vi "ParameterOptimizationCalibration.vi"() -> ()   [LabVIEW 2020]
uses:
  <vilib>/silver_ctls/ArrayMatrixCluster/Real Matrix NI_Silver.ctl
  <vilib>/gmath/GlobalOptimization.llb/DE_Settings.ctl
  <vilib>/gmath/GlobalOptimization.llb/DE_Bound Mapping Method.ctl
  <vilib>/gmath/GlobalOptimization.llb/DE_Mutation Method.ctl
  <vilib>/gmath/GlobalOptimization.llb/DE_Crossover Method.ctl
  <vilib>/gmath/GlobalOptimization.llb/DE_Stopping Criteria.ctl
  <vilib>/gmath/GlobalOptimization.llb/DE_State.ctl
  <vilib>/gmath/GlobalOptimization.llb/DE_Population.ctl
  <vilib>/gmath/NI_AAL_GlobalOptimization.lvlib
panel:
  out "number of function calls":i32
  out "Minimum":dbl[](array[numeric])
  out "F(Minimum)":dbl[](array[numeric])
  in  "Beginning State":T1
  in  "stopping criteria":T3={"max iterations"=50, "max function calls"=-1, "max time (sec)"=-1.0}
  in  "DE settings":T4={"population size"=10, "scale factor"=0.9, "crossover probability"=0.95, "bound mapping method"=1, "mutation method"=0, "crossover method"=0} {"crossover method" items=["Uniform", "Exponential"]; "mutation method" items=["Random", "Either Or", "Best", "Target to Best"]; "bound mapping method" items=["None", "Random between Bounds and Values", "Re-Initialize"]}
  out "min index(es)":i32[](array[numeric])
  out "min value":dbl
  out "Intensity Graph":dbl[][](graph)
  in  "P(x)":dbl[](array[numeric])=[-0.407, 0.781, 0.000845, -0.0056] step=1e-10 format="%#.8f"
  out "Real Matrix":T8
  in  "Offset (D)":dbl[](array[numeric])=[-0.4, -0.5, 2.0, 3.0, 4.0]
  in  "C parameter":dbl[](array[numeric])=[0.0, 1.0, 2.0, 3.0, 4.0]
  out "Measured":waveform(dbl)(graph)={"t0"=timestamp(0 s since 1904-01-01), "dt"=1.0, "Y"=array[3075 elements]}
  out "error":waveform(dbl)(graph)={"t0"=timestamp(0 s since 1904-01-01), "dt"=1.0, "Y"=array[3075 elements]}
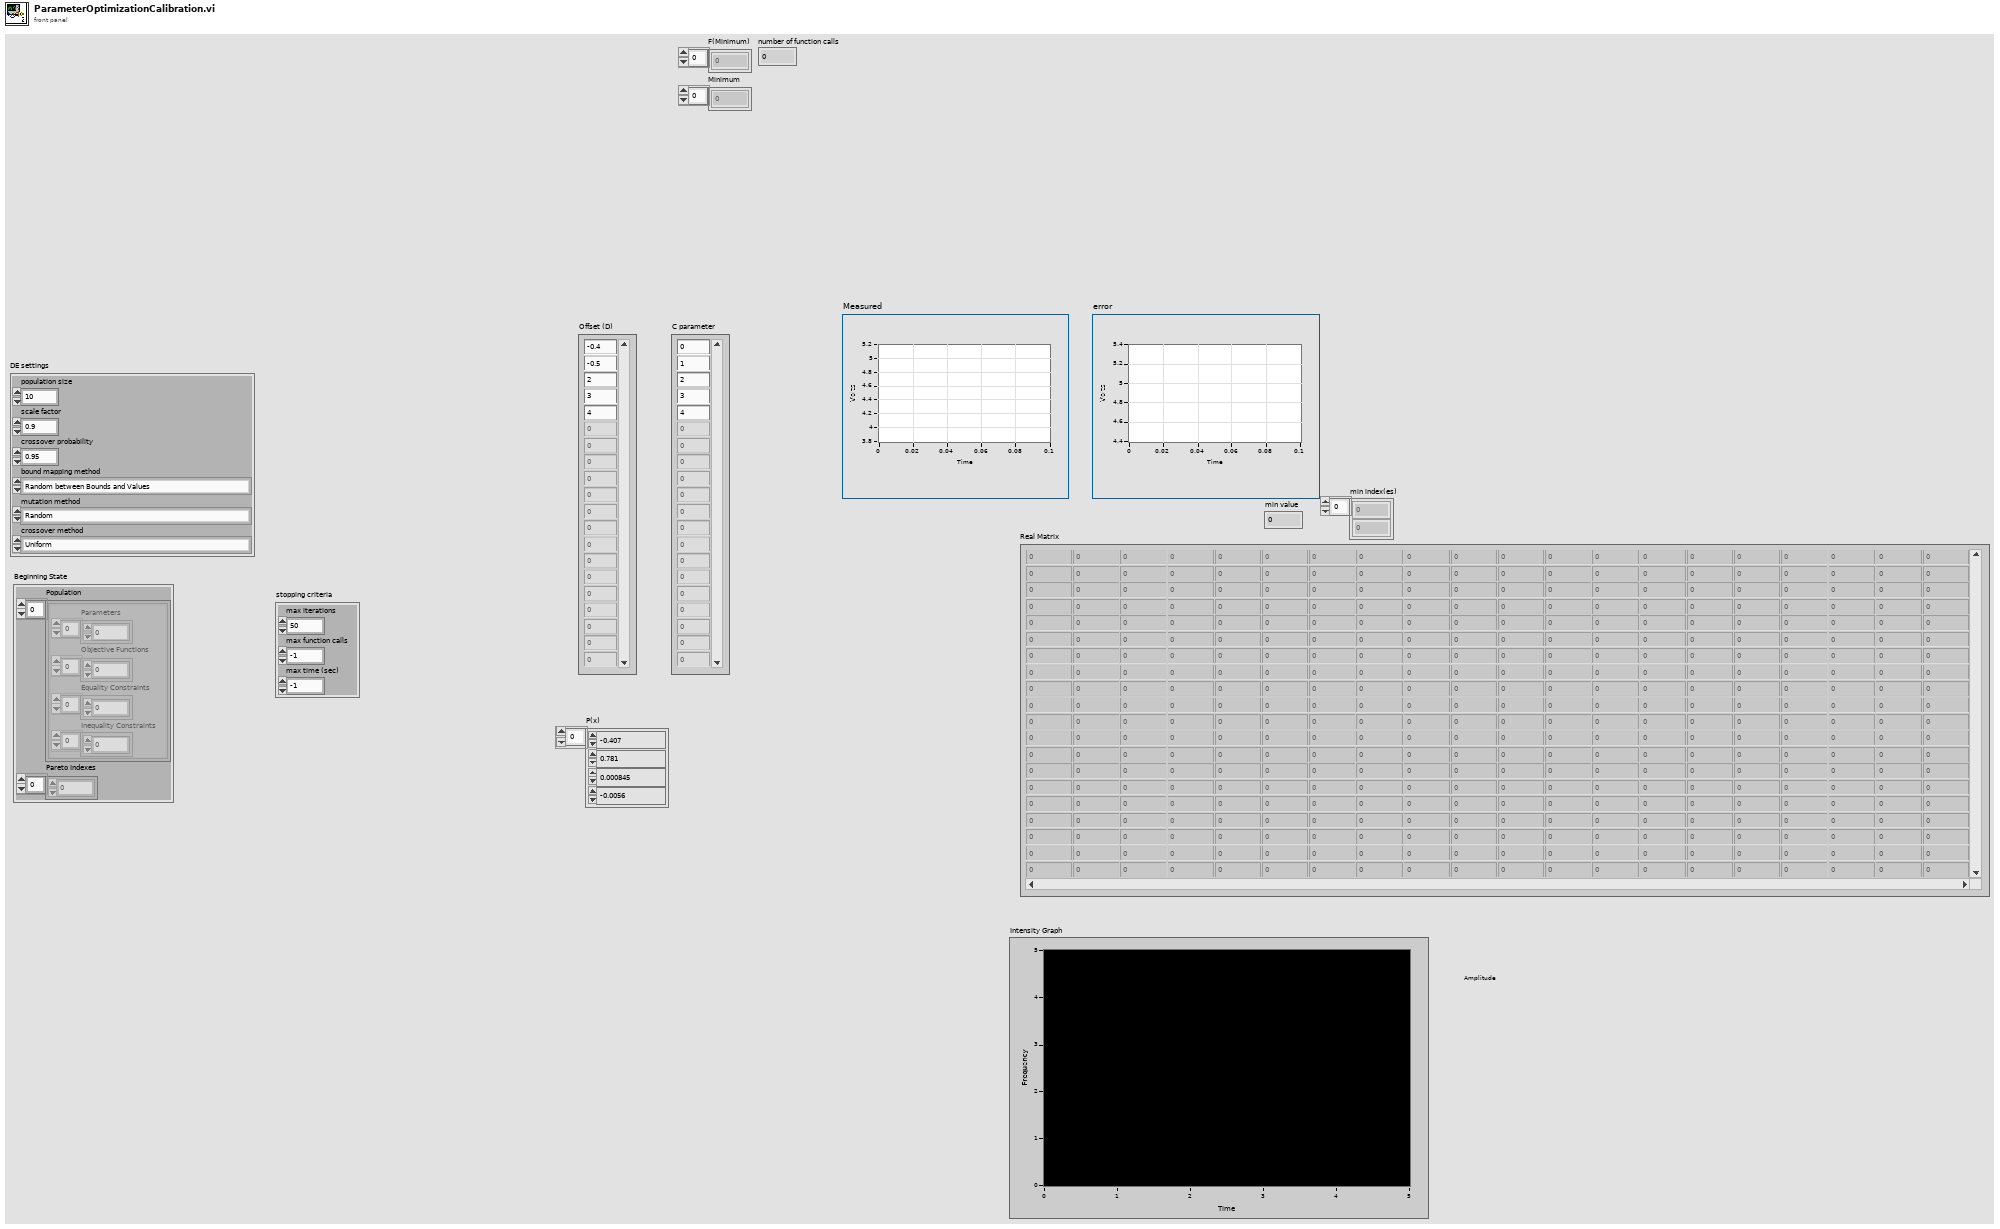
[diagram p1: front panel]
types:
  T1 = typedef "NI_AAL_GlobalOptimization.lvlib/DE_State.ctl" = cluster{"Population":T2[], "Pareto Indexes":i32[]}
  T2 = typedef "NI_AAL_GlobalOptimization.lvlib/DE_Population.ctl" = cluster{"Parameters":dbl[], "Objective Functions":dbl[], "Equality Constraints":dbl[], "Inequality Constraints":dbl[]}
  T3 = typedef "NI_AAL_GlobalOptimization.lvlib/DE_Stopping Criteria.ctl" = cluster{"max iterations":i32, "max function calls":i32, "max time (sec)":dbl}
  T4 = typedef "NI_AAL_GlobalOptimization.lvlib/DE_Settings.ctl" = cluster{"population size":i32, "scale factor":dbl, "crossover probability":dbl, "bound mapping method":T5, "mutation method":T6, "crossover method":T7}
  T5 = typedef "NI_AAL_GlobalOptimization.lvlib/DE_Bound Mapping Method.ctl" = u16
  T6 = typedef "NI_AAL_GlobalOptimization.lvlib/DE_Mutation Method.ctl" = u16
  T7 = typedef "NI_AAL_GlobalOptimization.lvlib/DE_Crossover Method.ctl" = u16
  T8 = typedef "Real Matrix NI_Silver.ctl" = dbl[][]
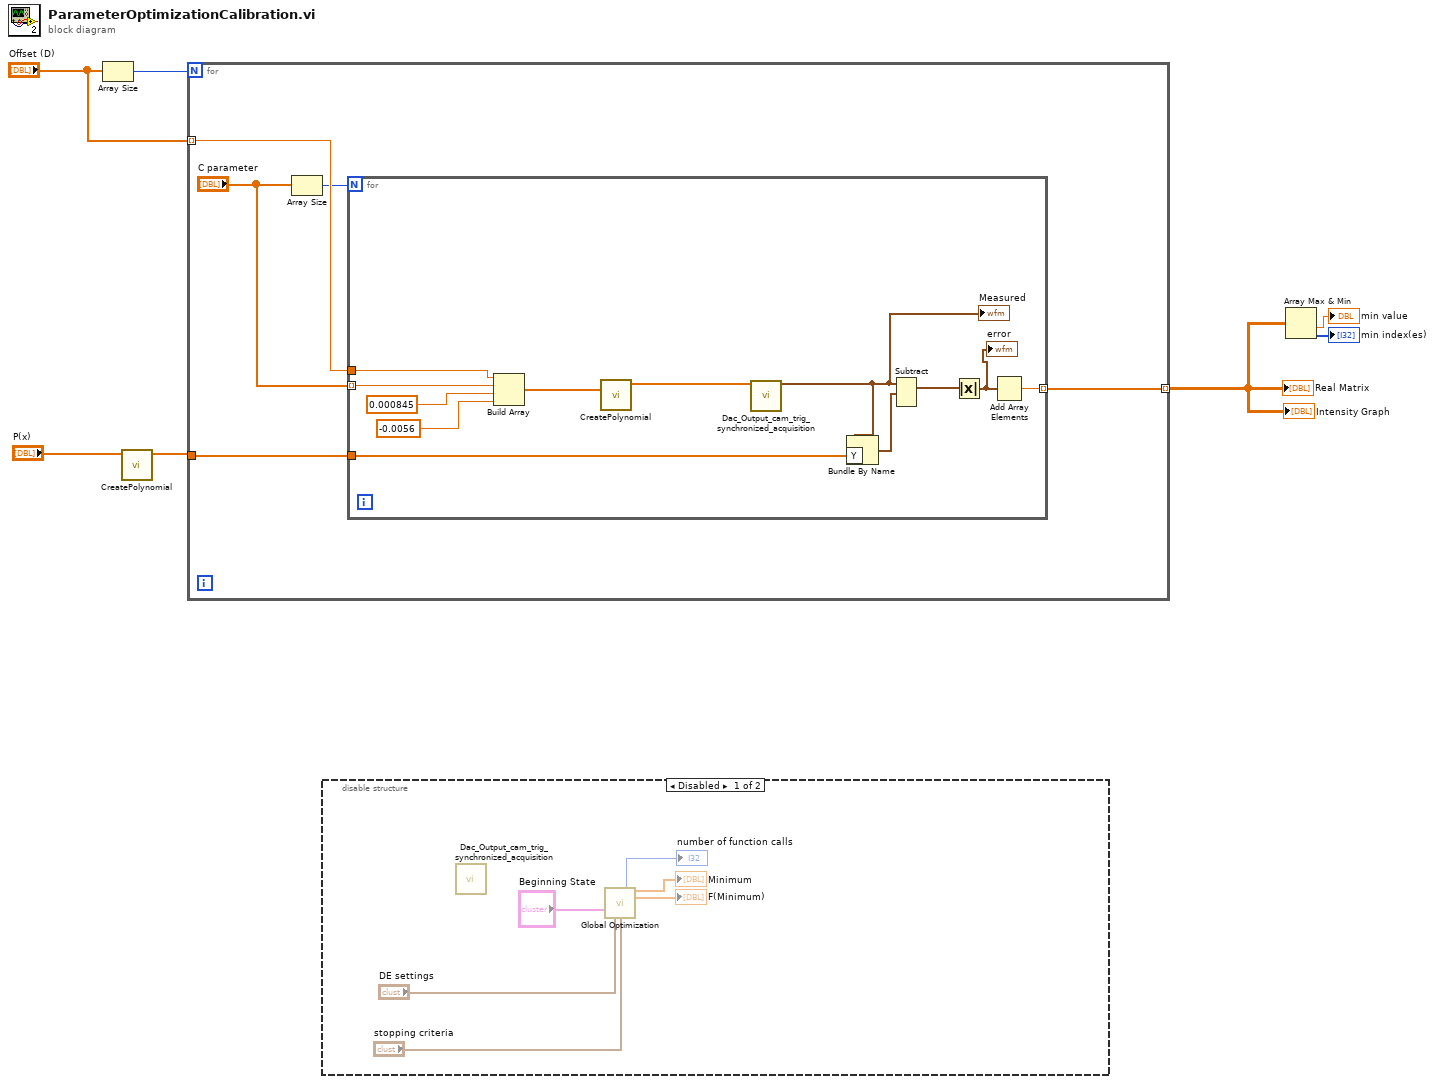
[diagram p0: block diagram]
diagram:
  n1 = Array Size(array="Offset (D)") -> (size(s)=w7:i32)
  n2 = call "CreatePolynomial.vi"("P(x)"="P(x)") -> ("Waveform Graph"=w4:dbl[])  [unwired: 9 in]
  n3 = for {
    N: w7 -> [_]
    tunnel: [w12] -> w3 mode=indexing
    tunnel: "Offset (D)" -> [w10] mode=indexing
    tunnel: w4 -> [w11]
    n4 = Array Size(array="C parameter") -> (size(s)=w9:i32)
    n5 = for {
      N: w9 -> [_]
      tunnel: [w24] -> w12 mode=indexing
      tunnel: w11 -> [w19]
      tunnel: "C parameter" -> [w14] mode=indexing
      tunnel: w10 -> [w13]
      n6 = Build Array(w13, w14, 0.000845 ("element"), -0.0056 ("element")) -> (w17:dbl[])
      n7 = call "CreatePolynomial.vi"("P(x)"=w17) -> ("Waveform Graph"=w18:dbl[])  [unwired: 9 in]
      n8 = call "Dac_Output_cam_trig_synchronized_acquisition.vi"("LabVIEW generated Sawtooth input"=w18) -> ("Measured voltage"=w20:waveform(dbl))  [unwired: 18 in]
      "Measured" <- w20
      n9 = Bundle By Name(cluster=w20, "Y"=w19) -> (w21:waveform(dbl))
      n10 = Subtract(1:w21, 2:w20) -> (0:w23:waveform(dbl))  [unwired: 1 in, 1 out]
      n11 = Absolute Value(x=w23) -> (abs(x)=w22:waveform(dbl))
      "error" <- w22
      n12 = Add Array Elements(numeric array=w22) -> (sum=w24:dbl)
    }
  }
  "Real Matrix" <- w3
  "Intensity Graph" <- w3
  n13 = disable-structure shown="Disabled" {
    frame Disabled {
      n14 = call "Dac_Output_cam_trig_synchronized_acquisition.vi"() -> ()  [unwired: 19 in, 1 out]
      n15 = call <vilib>:"Global Optimization.vi"("Beginning State"="Beginning State", "DE settings"="DE settings", "stopping criteria"="stopping criteria") -> ("number of function calls"=→"number of function calls":i32, "Minimum"=→"Minimum":dbl[], "F(Minimum)"=→"F(Minimum)":dbl[])  [unwired: 8 in, 2 out]
    }
    frame Enabled {
    }
  }
  n16 = Array Max & Min(array=w3) -> (min value=→"min value":dbl, min index (indices)=→"min index(es)":i32[])  [unwired: 2 out]
